vi "계산기 제작 최종.vi"() -> ()   [LabVIEW 2018]
panel:
  in  "취소 버튼":bool
  out "문자열":string
  in  "계산기":T1
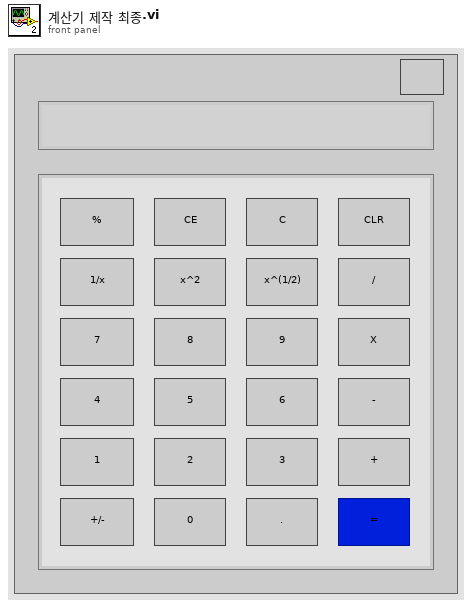
[diagram p1: front panel]
types:
  T1 = cluster{"%":bool, "CE":bool, "C":bool, "CLR":bool, "1/x":bool, "x^2":bool, "x^(1/2)":bool, "/":bool, "7":bool, "8":bool, "9":bool, "X":bool, "4":bool, "5":bool, "6":bool, "-":bool, "1":bool, "2":bool, "3":bool, "+":bool, "+/-":bool, "0":bool, ".":bool, "=":bool}
  T2 = enum16{"function", "plus", "minus", "multi", "division"}
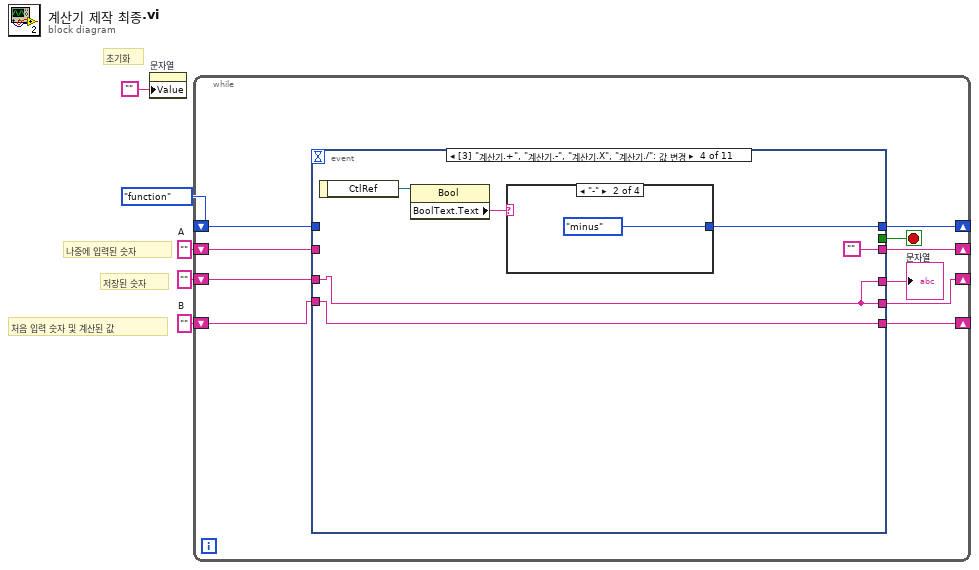
[diagram p0: block diagram]
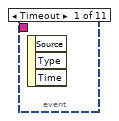
[diagram p2: hidden frame]
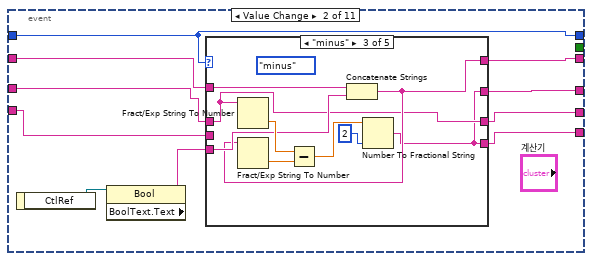
[diagram p3: hidden frame]
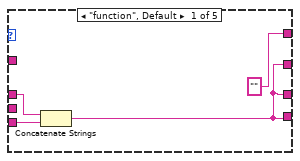
[diagram p4: hidden frame]
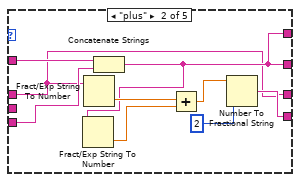
[diagram p5: hidden frame]
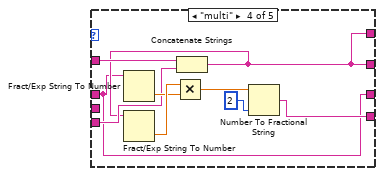
[diagram p6: hidden frame]
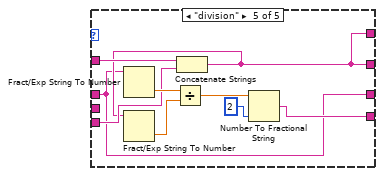
[diagram p7: hidden frame]
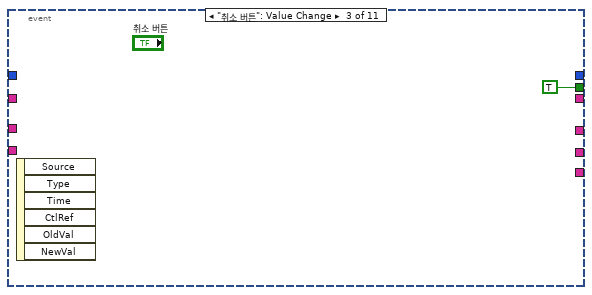
[diagram p8: hidden frame]
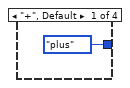
[diagram p9: hidden frame]
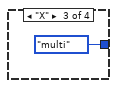
[diagram p10: hidden frame]
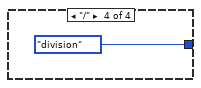
[diagram p11: hidden frame]
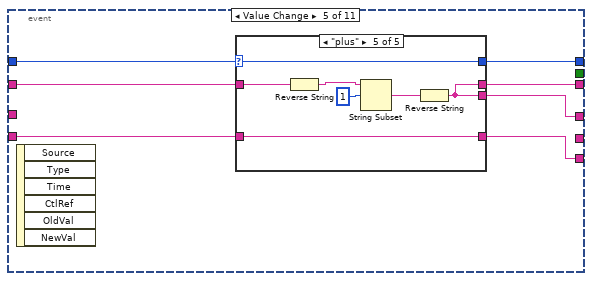
[diagram p12: hidden frame]
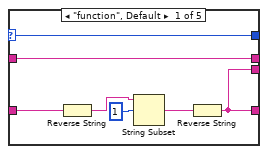
[diagram p13: hidden frame]
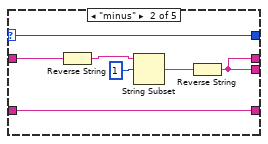
[diagram p14: hidden frame]
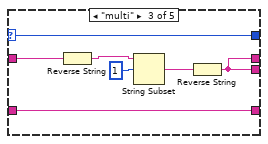
[diagram p15: hidden frame]
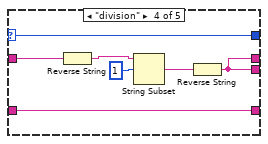
[diagram p16: hidden frame]
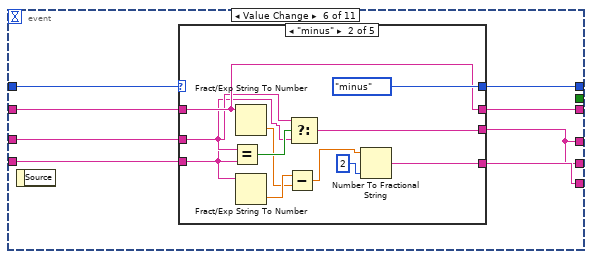
[diagram p17: hidden frame]
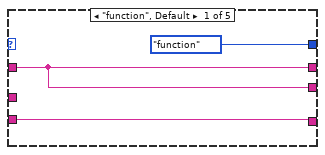
[diagram p18: hidden frame]
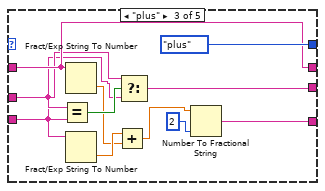
[diagram p19: hidden frame]
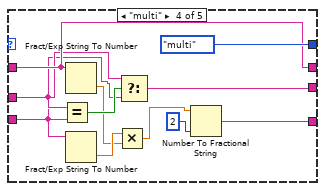
[diagram p20: hidden frame]
diagram:
  w4 = ""  # B
  w5 = ""  # A
  # "초기화"
  # "나중에 입력된 숫자"
  # "저장된 숫자"
  # "처음 입력 숫자 및 계산된 값"
  n1 = property on="문자열" class="Str"("Value"="") -> ()  [unwired: 2 in, 2 out]
  n2 = while {
    shift-right: [w8] -> _
    shift-left: w5 -> [w13]
    shift-right: [w9] -> _
    shift-left: w4 -> [w11]
    shift-right: [w14] -> _
    shift-left: T2."function" -> [w15]
    shift-right: [w7] -> _
    shift-left: "" -> [w6]
    stop <- w10 stop-if-true
    n3 = event shown="[3] \"계산기.+\", \"계산기.-\", \"계산기.X\", \"계산기./\": 값 변경" {
      selector: _ -> [_ _ _ _ _ _ _ _ _ _ _]
      dyn-events: _ -> [_ _ _ _ _ _ _ _ _ _ _]
      timeout: _ -> [_ _ _ _ _ _ _ _ _ _ _]
      tunnel: w15 -> [_ w21 _ _ w83 w126 _ _ _ _ _]
      tunnel: [_ w21 _ w70 w78 w123 T2."function" _ _ _ _] -> w14
      tunnel: w13 -> [_ w20 _ _ w80 w124 _ _ _ _ _]
      tunnel: [_ w22 _ "" w79 w122 "" _ _ _ _] -> w8
      tunnel: [_ w23 _ w67 w77 w119 "" w178 w182 w186 w191] -> w12
      tunnel: w11 -> [_ w17 _ w68 w82 w125 _ w179 w183 w187 w190]
      tunnel: [_ w18 _ w68 w81 w120 "" w178 w182 w186 w191] -> w9
      tunnel: [_ _ TRUE _ _ _ _ _ _ _ _] -> w10
      tunnel: [_ w16 _ w67 _ w119 _ _ _ _ _] -> w7
      tunnel: w6 -> [_ w19 _ w67 _ w121 _ _ _ _ _]
      event Timeout {
        n4 = event-data() -> ()  [unwired: 1 in, 3 out]
      }
      event "계산기.0", "계산기.1", "계산기.2", "계산기.3", "계산기.4", "계산기.5", "계산기.6", "계산기.7", "계산기.8", "계산기.9", "계산기..": Value Change {
        n5 = event-data() -> ("CtlRef"=w25:refnum<vi>)  [unwired: 1 in]
        n6 = property class="Bool"(reference=w25) -> ("BoolText.Text"=w24:string)  [unwired: 1 in, 2 out]
        n7 = case shown="\"minus\"" w21 {
          tunnel: w20 -> [_ w38 w47 w56 w65]
          tunnel: w24 -> [w28 w37 w42 w51 w59]
          tunnel: [w26 w31 w39 w50 w58] -> w23
          tunnel: ["" w31 w41 w50 w58] -> w22
          tunnel: w19 -> [w27 w30 w40 w48 w57]
          tunnel: [w26 w32 w39 w49 w60] -> w18
          tunnel: w17 -> [_ _ _ _ _]
          tunnel: [w26 w30 w40 w48 w57] -> w16
          frame "function", Default {
            n8 = Concatenate Strings(w27, w28) -> (w26:string)
          }
          frame "plus" {
            n9 = Fract/Exp String To Number(string=w30) -> (number=w35:dbl)  [unwired: 3 in, 1 out]
            n10 = Concatenate Strings(w38, w37) -> (w31:string)
            n11 = Fract/Exp String To Number(string=w31) -> (number=w34:dbl)  [unwired: 3 in, 1 out]
            n12 = Add(x=w35, y=w34) -> (x+y=w36:dbl)
            n13 = Number To Fractional String(number=w36, precision (6)=2) -> (F-format string=w32:string)  [unwired: 2 in]
          }
          frame "minus" {
            (unwired) T2."minus"
            n14 = Fract/Exp String To Number(string=w40) -> (number=w45:dbl)  [unwired: 3 in, 1 out]
            n15 = Concatenate Strings(w47, w42) -> (w41:string)
            n16 = Fract/Exp String To Number(string=w41) -> (number=w44:dbl)  [unwired: 3 in, 1 out]
            n17 = Subtract(x=w45, y=w44) -> (x-y=w46:dbl)
            n18 = Number To Fractional String(number=w46, precision (6)=2) -> (F-format string=w39:string)  [unwired: 2 in]
          }
          frame "multi" {
            n19 = Fract/Exp String To Number(string=w48) -> (number=w54:dbl)  [unwired: 3 in, 1 out]
            n20 = Concatenate Strings(w56, w51) -> (w50:string)
            n21 = Fract/Exp String To Number(string=w50) -> (number=w55:dbl)  [unwired: 3 in, 1 out]
            n22 = Multiply(x=w55, y=w54) -> (x*y=w53:dbl)
            n23 = Number To Fractional String(number=w53, precision (6)=2) -> (F-format string=w49:string)  [unwired: 2 in]
          }
          frame "division" {
            n24 = Fract/Exp String To Number(string=w57) -> (number=w62:dbl)  [unwired: 3 in, 1 out]
            n25 = Concatenate Strings(w65, w59) -> (w58:string)
            n26 = Fract/Exp String To Number(string=w58) -> (number=w63:dbl)  [unwired: 3 in, 1 out]
            n27 = Divide(x=w62, y=w63) -> (x/y=w64:dbl)
            n28 = Number To Fractional String(number=w64, precision (6)=2) -> (F-format string=w60:string)  [unwired: 2 in]
          }
        }
      }
      event "취소 버튼": Value Change {
        n29 = event-data() -> ()  [unwired: 1 in, 6 out]
      }
      event "계산기.+", "계산기.-", "계산기.X", "계산기./": Value Change {
        n30 = event-data() -> ("CtlRef"=w72:refnum<vi>)  [unwired: 1 in]
        n31 = property class="Bool"(reference=w72) -> ("BoolText.Text"=w71:string)  [unwired: 1 in, 2 out]
        n32 = case shown="\"-\"" w71 {
          tunnel: [T2."plus" T2."minus" T2."multi" T2."division"] -> w70
          frame "+", Default {
          }
          frame "-" {
          }
          frame "X" {
          }
          frame "/" {
          }
        }
      }
      event "계산기.CLR": Value Change {
        n33 = event-data() -> ()  [unwired: 1 in, 6 out]
        n34 = case shown="\"plus\"" w83 {
          selector: w83 -> [w85 w92 w99 w106 w113]
          tunnel: w82 -> [w88 w93 w100 w107 w114]
          tunnel: [w84 w93 w100 w107 w114] -> w81
          tunnel: w80 -> [w86 w94 w101 w108 w115]
          tunnel: [w86 w91 w98 w105 w112] -> w79
          tunnel: [w85 w92 w99 w106 w113] -> w78
          tunnel: [w84 w91 w98 w105 w112] -> w77
          frame "function", Default {
            n35 = Reverse String(1:w88) -> (0:w89:string)
            n36 = String Subset(string=w89, offset (0)=1) -> (substring=w90:string)  [unwired: 1 in]
            n37 = Reverse String(1:w90) -> (0:w84:string)
          }
          frame "minus" {
            n38 = Reverse String(1:w94) -> (0:w96:string)
            n39 = String Subset(string=w96, offset (0)=1) -> (substring=w97:string)  [unwired: 1 in]
            n40 = Reverse String(1:w97) -> (0:w91:string)
          }
          frame "multi" {
            n41 = Reverse String(1:w101) -> (0:w103:string)
            n42 = String Subset(string=w103, offset (0)=1) -> (substring=w104:string)  [unwired: 1 in]
            n43 = Reverse String(1:w104) -> (0:w98:string)
          }
          frame "division" {
            n44 = Reverse String(1:w108) -> (0:w110:string)
            n45 = String Subset(string=w110, offset (0)=1) -> (substring=w111:string)  [unwired: 1 in]
            n46 = Reverse String(1:w111) -> (0:w105:string)
          }
          frame "plus" {
            n47 = Reverse String(1:w115) -> (0:w117:string)
            n48 = String Subset(string=w117, offset (0)=1) -> (substring=w118:string)  [unwired: 1 in]
            n49 = Reverse String(1:w118) -> (0:w112:string)
          }
        }
      }
      event "계산기.=": Value Change {
        n50 = event-data() -> ()  [unwired: 1 in, 1 out]
        n51 = case shown="\"minus\"" w126 {
          tunnel: w125 -> [w129 w130 w141 w152 w163]
          tunnel: [w129 w132 w143 w154 w165] -> w120
          tunnel: w124 -> [w128 w133 w144 w155 w166]
          tunnel: [w128 w133 w144 w155 w166] -> w122
          tunnel: [w128 w138 w149 w160 w171] -> w119
          tunnel: [T2."function" T2."minus" T2."plus" T2."multi" T2."division"] -> w123
          tunnel: w121 -> [_ w131 w142 w153 w164]
          frame "function", Default {
          }
          frame "minus" {
            n52 = Equal?(x=w131, y=w130) -> (x = y?=w139:bool)
            n53 = Fract/Exp String To Number(string=w133) -> (number=w135:dbl)  [unwired: 3 in, 1 out]
            n54 = Fract/Exp String To Number(string=w130) -> (number=w136:dbl)  [unwired: 3 in, 1 out]
            n55 = Subtract(x=w136, y=w135) -> (x-y=w137:dbl)
            n56 = Select(t=w131, s=w139, f=w130) -> (s? t:f=w138:string)
            n57 = Number To Fractional String(number=w137, precision (6)=2) -> (F-format string=w132:string)  [unwired: 2 in]
          }
          frame "plus" {
            n58 = Equal?(x=w142, y=w141) -> (x = y?=w150:bool)
            n59 = Fract/Exp String To Number(string=w144) -> (number=w146:dbl)  [unwired: 3 in, 1 out]
            n60 = Fract/Exp String To Number(string=w141) -> (number=w147:dbl)  [unwired: 3 in, 1 out]
            n61 = Add(x=w147, y=w146) -> (x+y=w148:dbl)
            n62 = Select(t=w142, s=w150, f=w141) -> (s? t:f=w149:string)
            n63 = Number To Fractional String(number=w148, precision (6)=2) -> (F-format string=w143:string)  [unwired: 2 in]
          }
          frame "multi" {
            n64 = Equal?(x=w153, y=w152) -> (x = y?=w161:bool)
            n65 = Fract/Exp String To Number(string=w155) -> (number=w157:dbl)  [unwired: 3 in, 1 out]
            n66 = Fract/Exp String To Number(string=w152) -> (number=w158:dbl)  [unwired: 3 in, 1 out]
            n67 = Multiply(x=w158, y=w157) -> (x*y=w159:dbl)
            n68 = Select(t=w153, s=w161, f=w152) -> (s? t:f=w160:string)
            n69 = Number To Fractional String(number=w159, precision (6)=2) -> (F-format string=w154:string)  [unwired: 2 in]
          }
          frame "division" {
            n70 = Equal?(x=w164, y=w163) -> (x = y?=w172:bool)
            n71 = Fract/Exp String To Number(string=w166) -> (number=w168:dbl)  [unwired: 3 in, 1 out]
            n72 = Fract/Exp String To Number(string=w163) -> (number=w169:dbl)  [unwired: 3 in, 1 out]
            n73 = Divide(x=w169, y=w168) -> (x/y=w170:dbl)
            n74 = Select(t=w164, s=w172, f=w163) -> (s? t:f=w171:string)
            n75 = Number To Fractional String(number=w170, precision (6)=2) -> (F-format string=w165:string)  [unwired: 2 in]
          }
        }
      }
      event "계산기.C": Value Change {
        n76 = event-data() -> ()  [unwired: 1 in, 6 out]
      }
      event "계산기.x^2": Value Change {
        n77 = event-data() -> ()  [unwired: 1 in, 1 out]
        n78 = Decimal String To Number(string=w179) -> (number=w180:i32)  [unwired: 2 in, 1 out]
        n79 = Square(x=w180) -> (x^2=w181:i32)
        n80 = Number To Decimal String(number=w181) -> (decimal integer string=w178:string)  [unwired: 1 in]
      }
      event "계산기.x^(1/2)": Value Change {
        n81 = event-data() -> ()  [unwired: 1 in, 1 out]
        n82 = Decimal String To Number(string=w183) -> (number=w184:i32)  [unwired: 2 in, 1 out]
        n83 = Square Root(x=w184) -> (sqrt(x)=w185:dbl)
        n84 = Number To Decimal String(number=w185) -> (decimal integer string=w182:string)  [unwired: 1 in]
      }
      event "계산기.1/x": Value Change {
        n85 = event-data() -> ()  [unwired: 1 in, 1 out]
        n86 = Decimal String To Number(string=w187) -> (number=w188:i32)  [unwired: 2 in, 1 out]
        n87 = Reciprocal(x=w188) -> (1/x=w189:dbl)
        n88 = Number To Decimal String(number=w189) -> (decimal integer string=w186:string)  [unwired: 1 in]
      }
      event "계산기.+/-": Value Change {
        n89 = event-data() -> ()  [unwired: 1 in, 1 out]
        n90 = Decimal String To Number(string=w190) -> (number=w192:i32)  [unwired: 2 in, 1 out]
        n91 = Negate(x=w192) -> (-x=w193:i32)
        n92 = Number To Fractional String(number=w193) -> (F-format string=w191:string)  [unwired: 3 in]
      }
    }
    "문자열" <- w12
  }
